vi "RSZVB Acquire Fixture Compensation Sweep.vi"(7 "Ports (none)":i32[](array[numeric]), 8 "error in (no error)":errorcluster {"code" format="%.0x"}, 9 "Standard Type (0)":i32(ring) items=["Open", "Short"], 10 "Channel (1)":i32=1, 11 "VISA session":refnum<visa-resource-name>) -> (0 "error out":errorcluster {"code" format="%.0x"}, 3 "dup VISA session":refnum<visa-resource-name>)   [LabVIEW 2011]
doc: "Starts a fixture compensation sweep in order to acquire measurement data for a test fixture that has its inner conductor terminated with the selected standards. \n\nRemote-control command(s):\n[SENSe<Ch>:]CORRection:COLLect:FIXTure[:ACQuire] OPEN | SHORT,\n<port_no>{,<port_no>}"
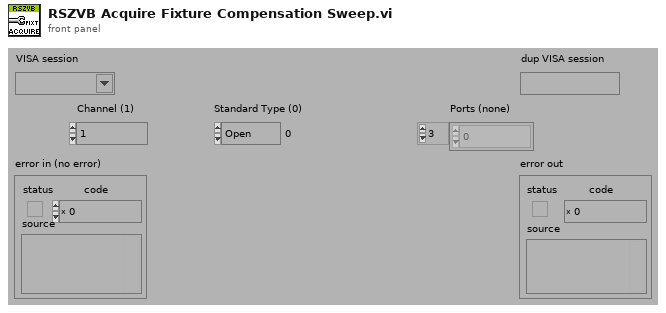
[diagram p1: front panel]
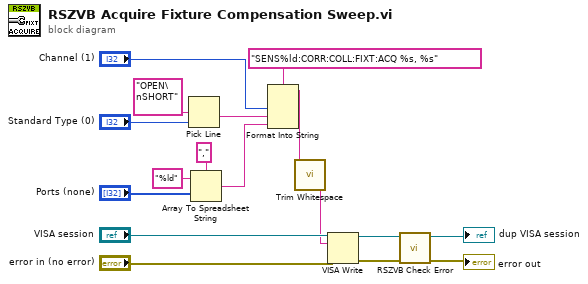
[diagram p0: block diagram]
diagram:
  n1 = Pick Line(multi-line string="OPEN\nSHORT", line index="Standard Type (0)") -> (output string=w10:string)  [unwired: 1 in]
  n2 = Array To Spreadsheet String(delimiter (Tab)=",", array="Ports (none)", 3:"%ld" ("format string")) -> (spreadsheet string=w9:string)
  n3 = Format Into String(format string="SENS%ld:CORR:COLL:FIXT:ACQ %s, %s", "Channel (1)", w10, w9) -> (resulting string=w6:string)  [unwired: 2 in, 1 out]
  n4 = call <vilib>:"Trim Whitespace.vi"("string"=w6) -> ("trimmed string"=w1:string)  [unwired: 1 in]
  n5 = VISA Write(VISA resource name="VISA session", write buffer=w1, error in (no error)="error in (no error)") -> (VISA resource name out=w3:refnum<visa-resource-name>, error out=w5:errorcluster)  [unwired: 1 out]
  n6 = call "RSZVB Check Error.vi"("error in (no error)"=w5, "VISA session"=w3) -> ("error out"=→"error out":errorcluster, "dup VISA session"=→"dup VISA session":refnum<visa-resource-name>)  [unwired: 8 in]
